vi "Frequency Set.vi"(6 "Update":bool=TRUE, 7 "Frequency":dbl format="%#_13g", 8 "error in (no error)":errorcluster, 9 "node":i32, 10 "idxChannel":i32, 11 "hdwf":i32) -> (0 "error out":errorcluster, 1 "func_out":i32, 5 "Frequency Out":dbl)   [LabVIEW 2024, in "AD2 DLL.lvlib"]
uses:
  AD2 DLL.lvlib
  <vilib>/Digilent/AD2 Toolkit/AD2.lvlib
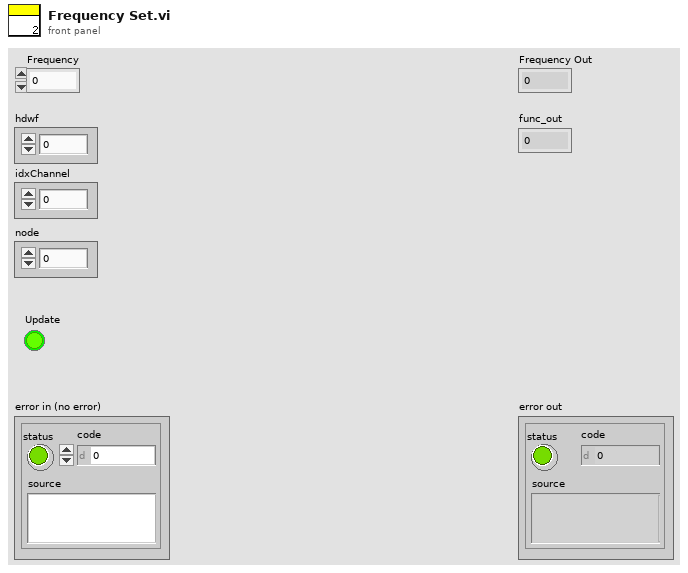
[diagram p1: front panel]
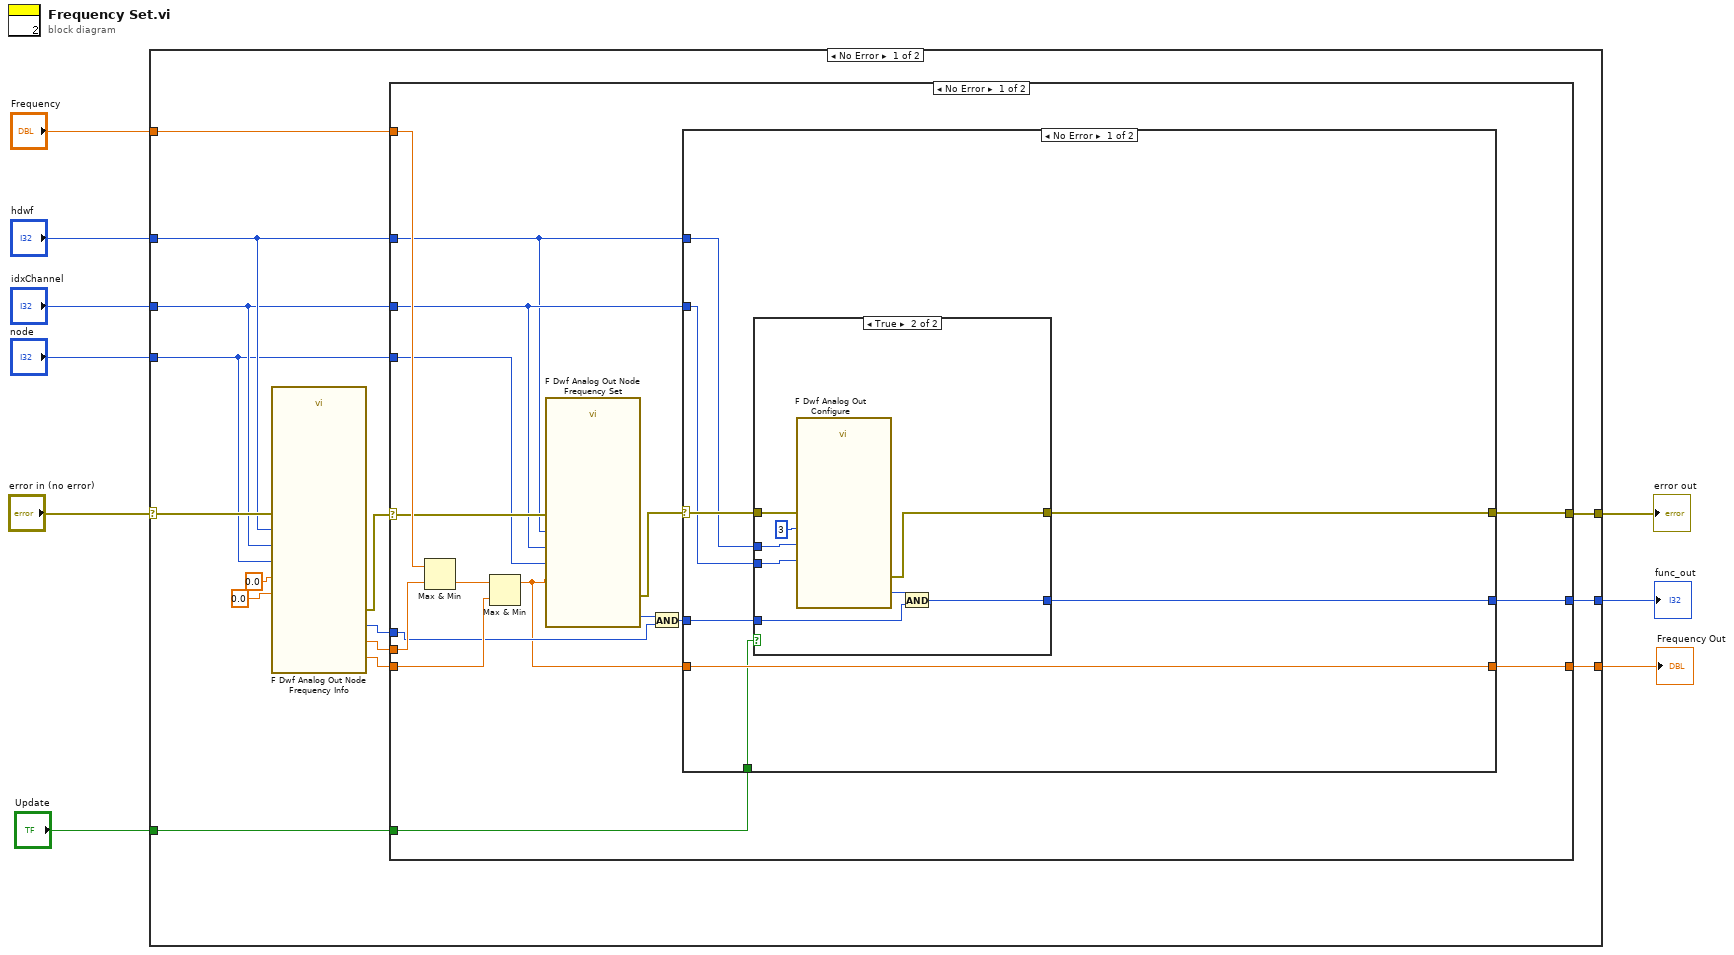
[diagram p0: block diagram]
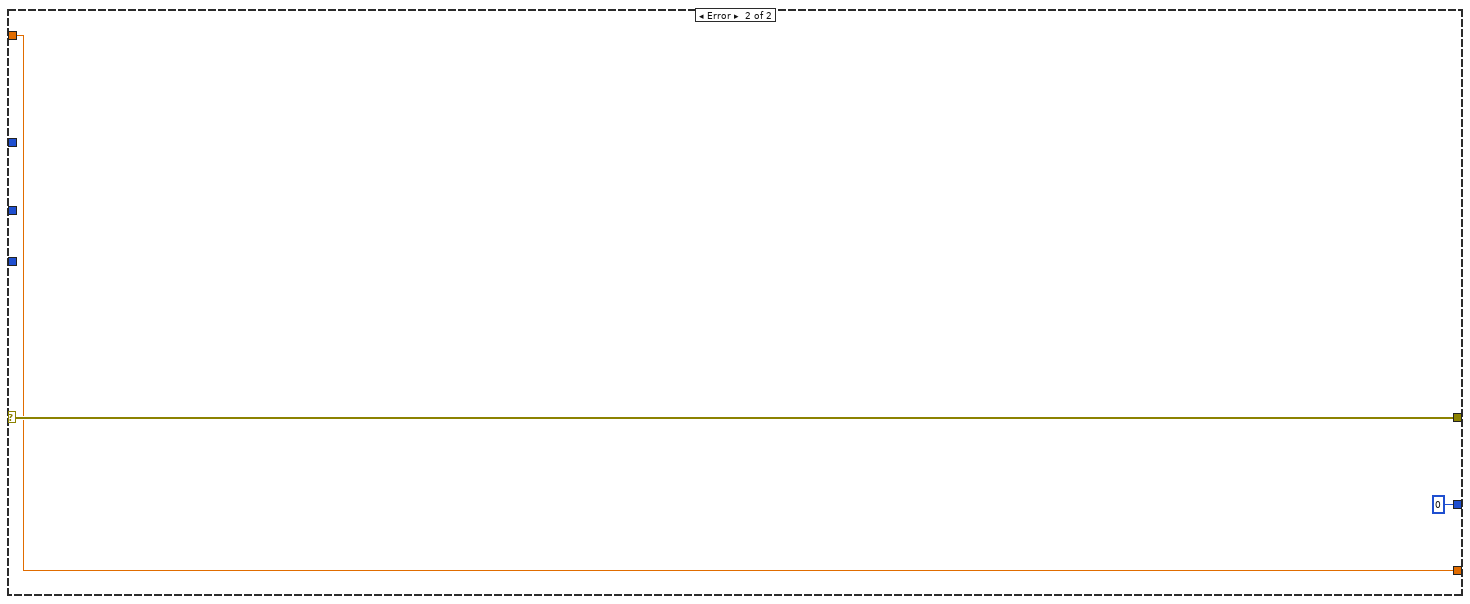
[diagram p5: hidden frame]
diagram:
  n1 = case shown="No Error" "error in (no error)" {
    selector: "error in (no error)" -> [w19 w68]
    tunnel: [w23 w68] -> w9
    tunnel: "hdwf" -> [w12 _]
    tunnel: "idxChannel" -> [w11 _]
    tunnel: "node" -> [w10 _]
    tunnel: "Frequency" -> [w24 w66]
    tunnel: [w22 0] -> w3
    tunnel: [w21 w66] -> w2
    tunnel: "Update" -> [w20 _]
    frame No Error {
      n2 = call <vilib>:"F Dwf Analog Out Node Frequency Info.vi"("phzMax"=0.0, "phzMin"=0.0, "error in (no error)"=w19, "node"=w10, "idxChannel"=w11, "hdwf"=w12) -> ("error out"=w18:errorcluster, "function return"=w17:i32, "phzMax out"=w16:dbl, "phzMin out"=w15:dbl)  [unwired: 2 in]
      n3 = case shown="No Error" w18 {
        selector: w18 -> [w30 w65]
        tunnel: w24 -> [w41 w63]
        tunnel: w16 -> [w40 _]
        tunnel: w15 -> [w38 _]
        tunnel: [w37 w65] -> w23
        tunnel: w12 -> [w25 _]
        tunnel: w11 -> [w27 _]
        tunnel: w10 -> [w26 _]
        tunnel: w17 -> [w36 w64]
        tunnel: [w34 w64] -> w22
        tunnel: [w33 w63] -> w21
        tunnel: w20 -> [w32 _]
        frame No Error {
          n4 = Max & Min(x=w41, y=w40) -> (min(x,y)=w39:dbl)  [unwired: 1 out]
          n5 = Max & Min(x=w39, y=w38) -> (max(x,y)=w29:dbl)  [unwired: 1 out]
          n6 = call <vilib>:"F Dwf Analog Out Node Frequency Set.vi"("hzFrequency"=w29, "error in (no error)"=w30, "node"=w26, "idxChannel"=w27, "hdwf"=w25) -> ("error out"=w31:errorcluster, "function return"=w28:i32)  [unwired: 5 in]
          n7 = And(x=w28, y=w36) -> (x .and. y?=w35:i32)
          n8 = case shown="No Error" w31 {
            selector: w31 -> [w49 w62]
            tunnel: [w46 w62] -> w37
            tunnel: w25 -> [w48 _]
            tunnel: w27 -> [w47 _]
            tunnel: w35 -> [w45 w61]
            tunnel: [w44 w61] -> w34
            tunnel: w29 -> [w43 w60]
            tunnel: [w43 w60] -> w33
            tunnel: w32 -> [w42 _]
            frame No Error {
              n9 = case shown="True" w42 {
                tunnel: w49 -> [w51 w59]
                tunnel: w48 -> [_ w57]
                tunnel: w47 -> [_ w56]
                tunnel: [w51 w55] -> w46
                tunnel: w45 -> [w50 w53]
                tunnel: [w50 w52] -> w44
                frame False {
                }
                frame True {
                  n10 = call <vilib>:"F Dwf Analog Out Configure.vi"("error in (no error)"=w59, "fStart"=3, "idxChannel"=w56, "hdwf"=w57) -> ("error out"=w55:errorcluster, "function return"=w54:i32)  [unwired: 6 in]
                  n11 = And(x=w54, y=w53) -> (x .and. y?=w52:i32)
                }
              }
            }
            frame Error {
            }
          }
        }
        frame Error {
        }
      }
    }
    frame Error {
    }
  }
  "error out" <- w9
  "func_out" <- w3
  "Frequency Out" <- w2
